vi "AFM_Driver_Manager.CreateWatchdogEvents.vi"(8 "error in (no error)":errorcluster, 11 "AFM_Driver_Manager in":refnum<class "AFM_Driver_Manager.lvclass">) -> (0 "error out":errorcluster, 3 "AFM_Driver_Manager out":refnum<class "AFM_Driver_Manager.lvclass">)   [LabVIEW 2020, in "AFM_Driver_Manager.lvclass"]
uses:
  AFM_Driver_Manager.lvclass
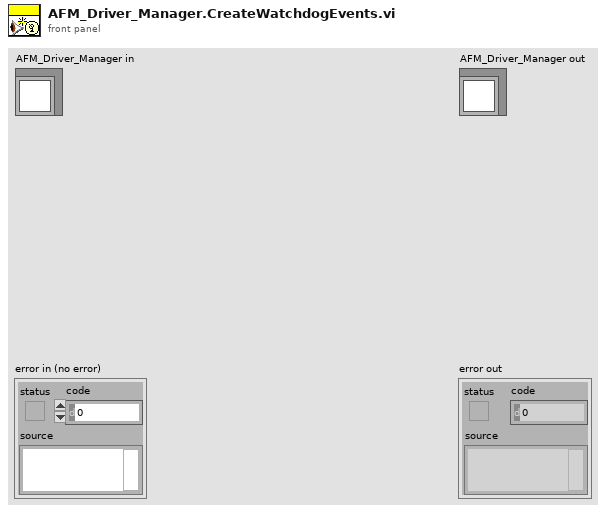
[diagram p1: front panel]
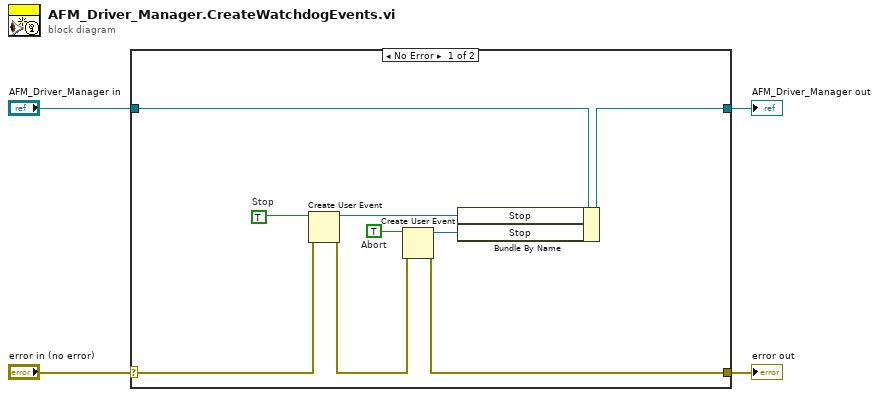
[diagram p0: block diagram]
diagram:
  n1 = case shown="No Error" "error in (no error)" {
    selector: "error in (no error)" -> [w12 w15]
    tunnel: [w5 w15] -> w3
    tunnel: [w11 w14] -> w1
    tunnel: "AFM_Driver_Manager in" -> [w10 w14]
    frame No Error {
      w8 = TRUE  # Abort
      w13 = TRUE  # Stop
      n2 = Create User Event(user event datatype=w13, error in=w12) -> (user event=w9:refnum<user-event>, error out=w6:errorcluster)
      n3 = Create User Event(user event datatype=w8, error in=w6) -> (user event=w7:refnum<user-event>, error out=w5:errorcluster)
      n4 = Bundle By Name(cluster=w10, "Stop"=w9, "Stop"=w7) -> (w11:refnum<class "AFM_Driver_Manager.lvclass">)
    }
    frame Error {
    }
  }
  "error out" <- w3
  "AFM_Driver_Manager out" <- w1
